vi "Send Data to DAQ.vi"(7 "Detector Manager":refnum<class "Detector Manager.lvclass">, 8 "error in (no error)":errorcluster, 9 "Channel":u16, 10 "Conditioned Data":variant, 11 "Father Of All Detectors in":refnum<class "Father Of All Detectors.lvclass">) -> (0 "error out":errorcluster, 3 "Father Of All Detectors out":refnum<class "Father Of All Detectors.lvclass">)   [LabVIEW 2026, in "TALOS.lvlib" / "Father Of All Detectors.lvlib" / "Father Of All Detectors.lvclass"]
uses:
  Father Of All Detectors.lvclass
  C:/LabVIEW Code/TALOS/talos/Classes/Hardware/Hardware.lvclass
  Internal uServices/System uServices/Detector Manager/Detector Manager/Detector Manager.lvclass
  C:/LabVIEW Code/TALOS/talos/Father of all uServices/Father of all uServices/Father of all uServices.lvclass
  Ancestor/Ancestor/Ancestor.lvclass/Ancestor.ctl
  Guardian/Guardian Messages/Message to uService Msg/Message to uService Msg.lvclass/Message to uService Msg.ctl
  <vilib>/AdvancedString/Delimited String to 1D String Array.vi
  <vilib>/AdvancedString/Delimited String to 1D String Array (string).vi
  Father of all uServices/Father of all uServices/Children Methods/Message to uService.vi
  Ancestor/Ancestor/Read ID.vi
  Guardian/Guardian Messages/Message to uService Msg/Send Message to uService.vi
  Support VIs/Substitute Error.vi
  Support VIs/Generate Error.vi
  FGV/Error Memory/Get Error Description.vi
  Support VIs/Get PC name.vi
  <vilib>/Utility/error.llb/Clear Errors.vi
  FGV/Error Memory/Error Memory Core.vi
  Support VIs/Circus Root Path.vi
  FGV/Error Memory/Error Crt Lvl checker.vi
  FGV/Error Memory/Error Memory Core.vi/40c8088d-b597-4017-91af-faa98e00292e.vi
  FGV/Error Memory/Error Memory Core.vi/d4a3ab98-063c-4e44-b43d-fbdcfe6c2be2.vi
  Father of all uServices/Father of all uServices/Father of all uServices.lvclass
  C:/LabVIEW Code/TALOS/talos/Ancestor/Ancestor/Ancestor.lvclass
  C:/LabVIEW Code/TALOS/builds/Actor Framework PPL/Actor Framework.lvlibp/1abvi3w/vi.lib/ActorFramework/Actor/Actor.lvclass
  <vilib>/Utility/LVClass/Get LV Class Name.vi
  Support VIs/Global Memory.vi
  builds/Actor Framework PPL/Actor Framework.lvlibp/1abvi3w/vi.lib/ActorFramework/Actor/Read Caller Enqueuer.vi
  builds/Actor Framework PPL/Actor Framework.lvlibp/1abvi3w/vi.lib/ActorFramework/Message Enqueuer/Enqueue.vi
  Support VIs/Is in Packed Library.vi
  Support VIs/TALOS Root path.vi
  Support VIs/Read CSV worksheet.vi
  Support VIs/Global Constants.vi
  <vilib>/Utility/error.llb/General Error Handler.vi
  Support VIs/Error Log.vi
  Guardian/Guardian Messages/Message to uService Msg/Message to uService Msg.lvclass
  Ancestor/Ancestor/Ancestor.lvclass
  <vilib>/Comparison/Equal/Equal Functor/Equal Functor.lvclass
  TALOS.lvlib
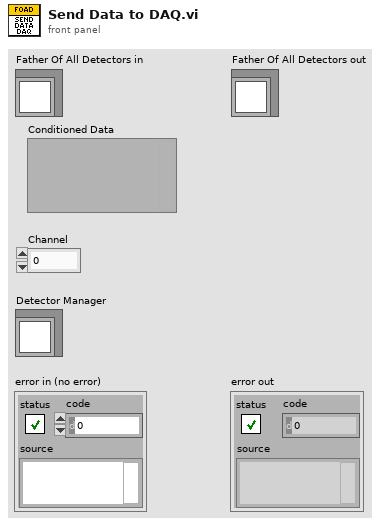
[diagram p1: front panel]
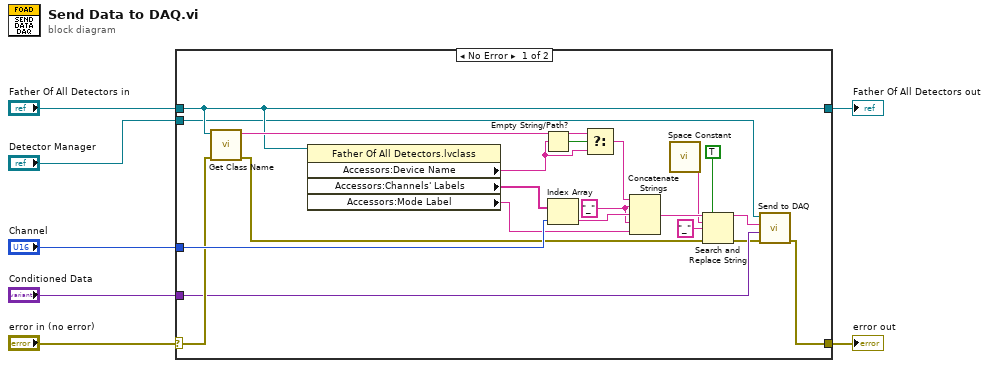
[diagram p0: block diagram]
diagram:
  n1 = case shown="No Error" "error in (no error)" {
    selector: "error in (no error)" -> [w25 w30]
    tunnel: [w9 w30] -> w6
    tunnel: [w17 w29] -> w4
    tunnel: "Father Of All Detectors in" -> [w17 w29]
    tunnel: "Channel" -> [w28 _]
    tunnel: "Conditioned Data" -> [w11 _]
    tunnel: "Detector Manager" -> [w8 _]
    frame No Error {
      w26 = "_" ("input 2")
      n2 = call "Get Class Name.vi"("error in (no error)"=w25, "object"=w17) -> ("error out"=w16:errorcluster, "Class Name"=w20:string)  [unwired: 8 in]
      n3 = property class="Father Of All Detectors.lvclass"(reference=w17) -> ("Accessors:Device Name"=w15:string, "Accessors:Channels' Labels"=w14:string[], "Accessors:Mode Label"=w13:string)  [unwired: 1 in, 2 out]
      n4 = Empty String/Path?(string/path=w15) -> (empty?=w19:bool)
      n5 = Index Array(array=w14, index=w28) -> (element=w27:string)
      n6 = Select(t=w20, s=w19, f=w15) -> (s? t:f=w18:string)
      n7 = Concatenate Strings(w18, w26, w27, w26, w13) -> (w24:string)
      n8 = call <vilib>:"Space Constant.vi"() -> ("String"=w22:string)
      n9 = Search and Replace String(replace all?=TRUE ("replace all? (F)"), input string=w24, search string=w22, replace string="_" ("replace string (\"\")"), error in=w16) -> (result string=w12:string, error out=w10:errorcluster)  [unwired: 3 in, 2 out]
      n10 = call "Send to DAQ.vi"("error in (no error)"=w10, "Data"=w11, "Data Name"=w12, "Father of all uServices in"=w8) -> ("error out"=w9:errorcluster)  [unwired: 6 in, 1 out]
    }
    frame Error {
    }
  }
  "error out" <- w6
  "Father Of All Detectors out" <- w4
